vi "Generate Json FileName.vi"(8 "error in (no error)":errorcluster, 11 "UIActorTop in":refnum<class "UIActorTop.lvclass">) -> (0 "error out":errorcluster, 2 "Json File path":path, 3 "UIActorTop out":refnum<class "UIActorTop.lvclass">)   [LabVIEW 2021, in "AbstractActorTemplate.lvlib" / "UIActorTop.lvclass"]
uses:
  <userlib>/John_Lib/AbstractActorTemplate/AbstractActorTemplate/UIActorTop.lvclass
  <userlib>/John_Lib/AbstractActorTemplate/AbstractActorTemplate/UIActorTop.lvclass/UIActorTop.ctl
  <userlib>/John_Lib/TopPath/TopPath.lvlib
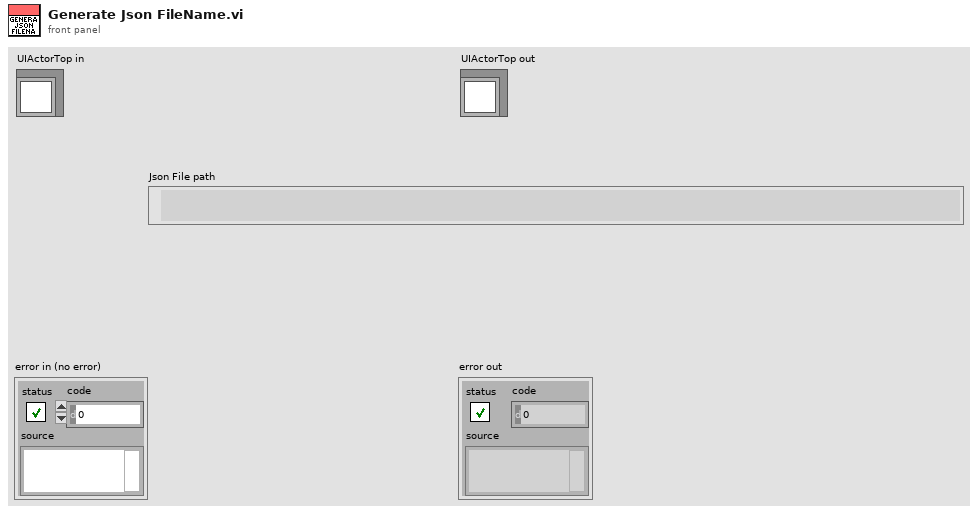
[diagram p1: front panel]
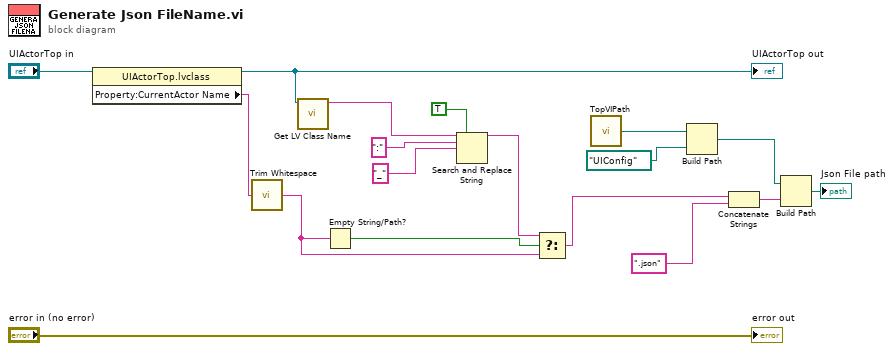
[diagram p0: block diagram]
diagram:
  n1 = property class="UIActorTop.lvclass"(reference="UIActorTop in") -> (reference out=w10:refnum<class "UIActorTop.lvclass">, "Property:CurrentActor Name"=w9:string)  [unwired: 1 in, 1 out]
  "UIActorTop out" <- w10
  n2 = call <vilib>:"Trim Whitespace.vi"("string"=w9) -> ("trimmed string"=w2:string)  [unwired: 1 in]
  n3 = call <vilib>:"Get LV Class Name.vi"("object"=w10) -> ("class name"=w5:string)  [unwired: 9 in, 1 out]
  n4 = Empty String/Path?(string/path=w2) -> (empty?=w4:bool)
  n5 = Search and Replace String(replace all?=TRUE ("replace all? (F)"), input string=w5, search string=":", replace string="_" ("replace string (\"\")")) -> (result string=w3:string)  [unwired: 4 in, 3 out]
  n6 = Select(t=w3, s=w4, f=w2) -> (s? t:f=w1:string)
  n7 = call <userlib>:"TopVIPath.vi"() -> ("ConfigFile path"=w12:path)  [unwired: 2 out]
  n8 = Build Path(base path=w12, name or relative path=path "UIConfig") -> (appended path=w15:path)
  n9 = Concatenate Strings(w1, ".json" ("string")) -> (w16:string)
  n10 = Build Path(base path=w15, name or relative path=w16) -> (appended path=→"Json File path":path)
  "error out" <- "error in (no error)"
